vi "LEP_RV_PrepareLaunch.vi"(8 "error in (no error)":errorcluster, 10 "Enable debugging":bool, 11 "Commands":T1) -> (0 "error out":errorcluster, 2 "debug occurrence":refnum<k4>, 3 "output cluster":refnum<vi>)   [LabVIEW 2011]
doc: "Download and execute built VxWorks downloadable module and attach the LabVIEW Embedded debuger."
uses:
  LEP_RV_Commands.ctl
  <vilib>/Platform/EmbProject/utilities/Emb_Utility_AppAction.ctl
  LEP_RV_Config.ctl
panel:
  out "output cluster 2":T4 {"Config"."Constant Deallocation" items=["Out of Scope", "VI End", "Application End"]; "Config"."Constant Allocation" items=["First Use", "Containing Loop", "VI Initialization", "Application Initialization"]; "Config"."Target serial port" items=["0", "1", "2", "3"]; "Config"."Console output" items=["Processor status window", "Serial port"]; "Config"."Optimization" items=["Level 0 (-O0)", "Level 1 (-O1)", "Level 2 (-O2)", "Level 3 (-O3)"]; "Config"."Mode" items=["ARM-Mode", "Thumb-Mode"]; "Config"."Debug Options" items=["Use ULINK Debugger", "Use Simulator"]; "Config"."Debug Mode" items=["Instrumented (serial port)", "Instrumented (TCP/IP)", "Non-instrumented (JTAG/USB)"]}
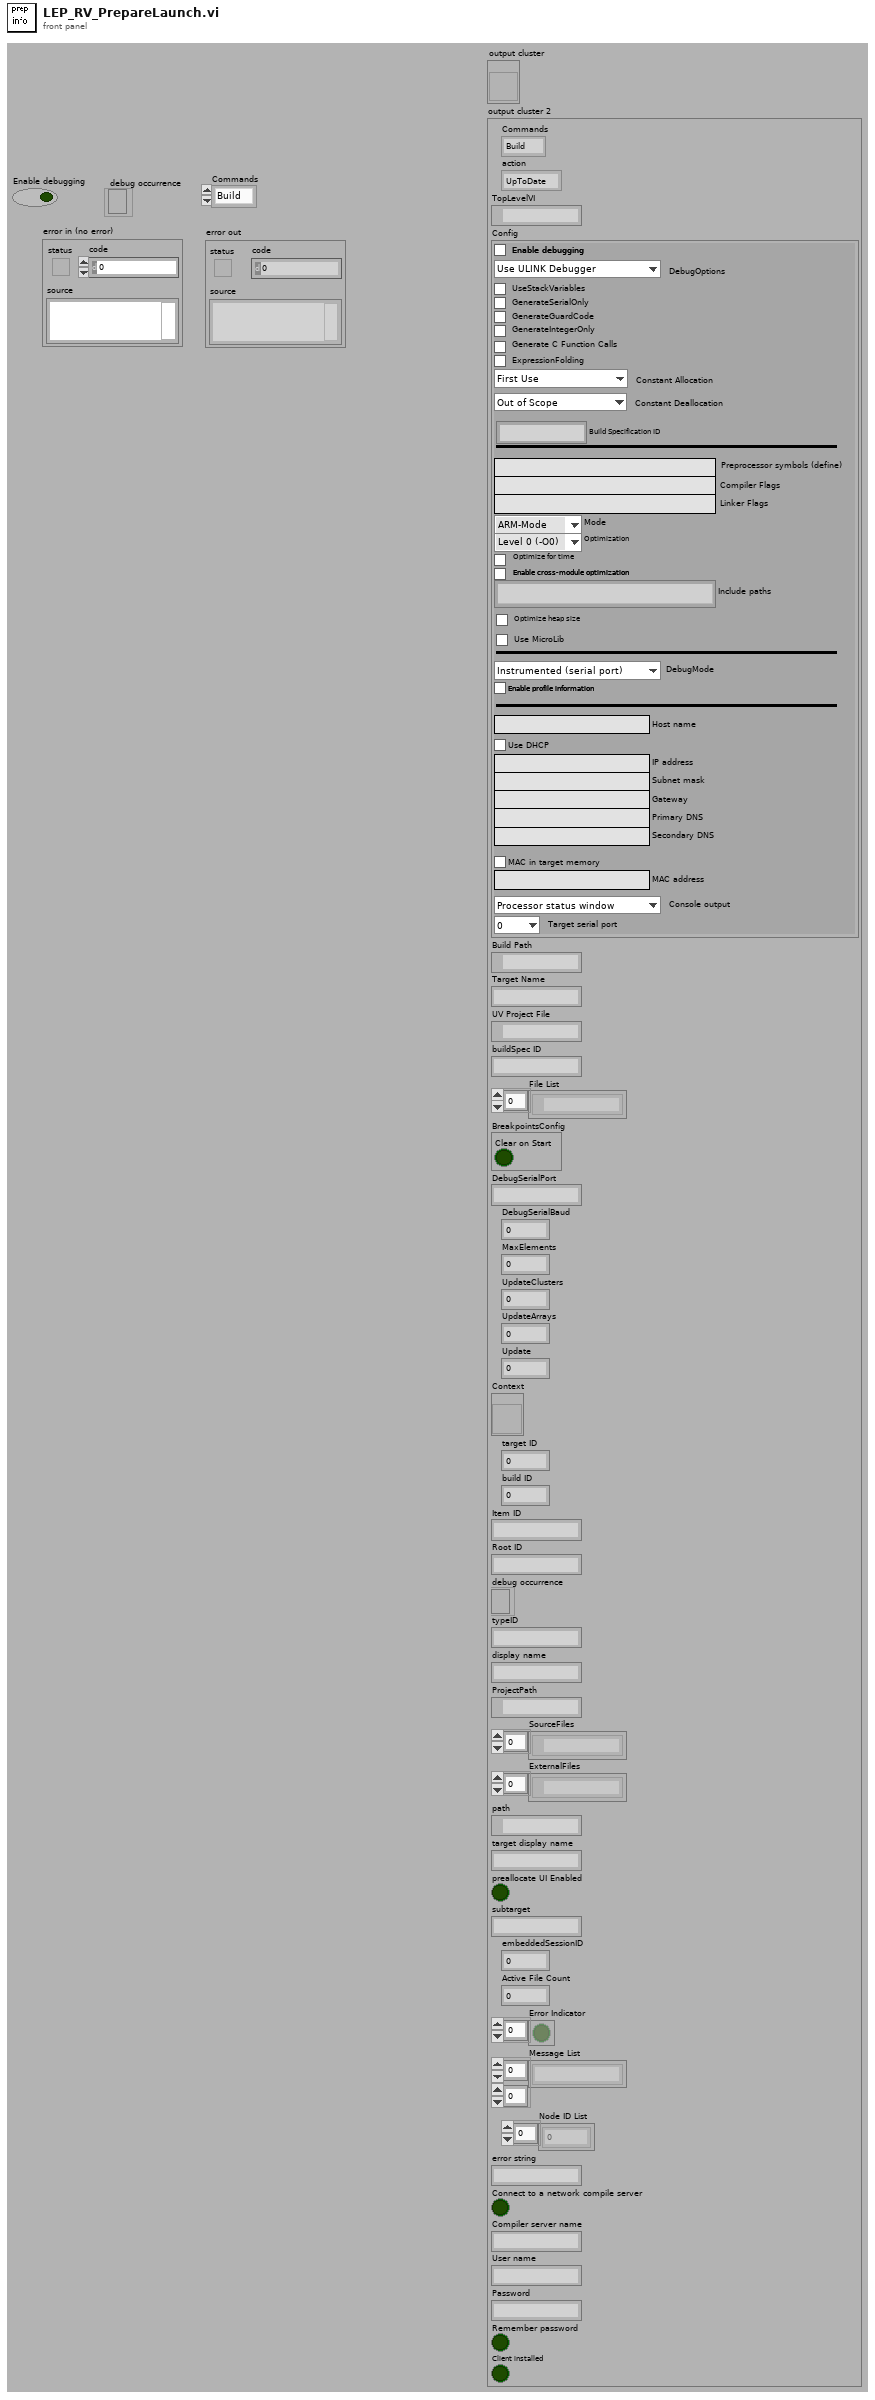
[diagram p1: front panel]
types:
  T1 = typedef "LEP_RV_Commands.ctl" = enum16{"Build", "Rebuild", "Run", "Debug", "Profile"}
  T2 = typedef "Emb_Utility_AppAction.ctl" = enum16{"UpToDate", "Build", "Cancel", "Error"}
  T3 = typedef "LEP_RV_Config.ctl" = cluster{"Enable debugging":bool, "Debug Options":u16, "Use stack variables":bool, "Generate serial only":bool, "Generate guard code":bool, "Generate Integer Only":bool, "Generate C Function Calls":bool, "ExpressionFolding":bool, "Constant Allocation":u16, "Constant Deallocation":u16, "Build Specification ID":string, "Preprocessor symbols (define)":string, "Compiler Flags":string, "Linker Flags":string, "Mode":u16, "Optimization":u16, "Optimize for time":bool, "Enable cross-module optimization":bool, "Include paths":path[], "Optimize heap size":bool, "Use MicroLib":bool, "Debug Mode":u16, "Enable profile information":bool, "Host name":string, "Use DHCP":bool, "IP address":string, "Subnet mask":string, "Gateway":string, "Primary DNS":string, "Secondary DNS":string, "MAC in target memory":bool, "MAC address":string, "Console output":u16, "Target serial port":u16}
  T4 = cluster{"Commands":T1, "action":T2, "TopLevelVI":path, "Config":T3, "Build Path":path, "Target Name":string, "UV Project File":path, "buildSpec ID":string, "File List":path[], "BreakpointsConfig":cluster{"Clear on Start":bool}, "DebugSerialPort":string, "DebugSerialBaud":u32, "MaxElements":u32, "UpdateClusters":u32, "UpdateArrays":u32, "Update":u32, "Context":refnum<vi>, "target ID":u32, "build ID":u32, "Item ID":string, "Root ID":string, "debug occurrence":refnum<k4>, "typeID":string, "display name":string, "ProjectPath":path, "SourceFiles":path[], "ExternalFiles":path[], "path":path, "target display name":string, "preallocate UI Enabled":bool, "subtarget":string, "embeddedSessionID":u32, "Active File Count":i32, "Error Indicator":bool[], "Message List":string[][], "Node ID List":i32[], "error string":string, "Connect to a network compile server":bool, "Compiler server name":string, "User name":string, "Password":string, "Remember password":bool, "Client installed":bool}
  T5 = enum16{"NoErr", "TopLevelVIErr", "EmptyTopLevelVIPath", "CGenErr", "CpySuppFilesErr", "ProjectInfoErr", "NoTopLevelVIErr", "CreateBuildFolderErr", "EmptyBuildFolderErr", "LoadConfigErr", "BildToolsErr", "CompileErr", "LinkError", "DebugInfoErr", "NotFoundErr", "AccessErr", "ExecErr", "UnknownErr"}
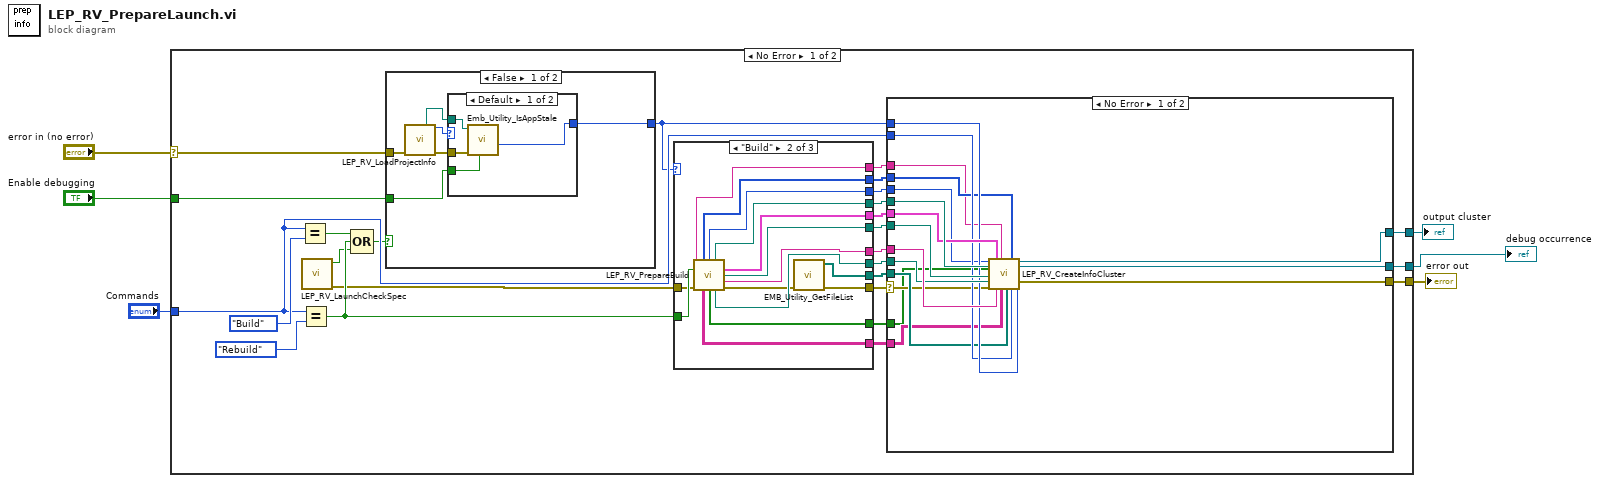
[diagram p0: block diagram]
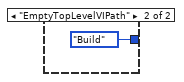
[diagram p2: hidden frame]
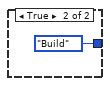
[diagram p3: hidden frame]
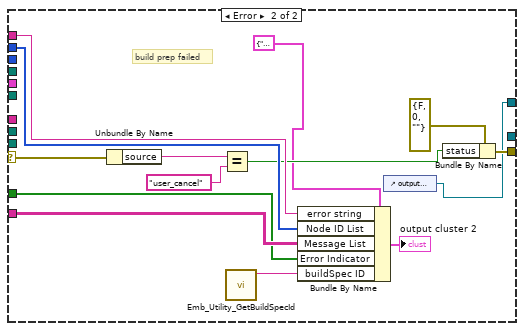
[diagram p4: hidden frame]
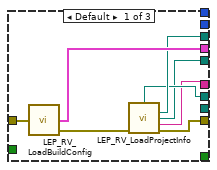
[diagram p5: hidden frame]
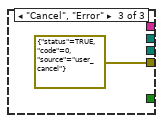
[diagram p6: hidden frame]
diagram:
  n1 = case shown="No Error" "error in (no error)" {
    selector: "error in (no error)" -> [w18 w100]
    tunnel: [w17 w100] -> w6
    tunnel: "Commands" -> [w30 _]
    tunnel: [w16 _] -> w3
    tunnel: "Enable debugging" -> [w15 _]
    tunnel: [w14 _] -> w1
    frame No Error {
      n2 = Equal?(x=w30, y=LEP_RV_Commands."Build") -> (x = y?=w27:bool)
      n3 = Equal?(x=w30, y=LEP_RV_Commands."Rebuild") -> (x = y?=w26:bool)
      n4 = call "LEP_RV_LaunchCheckSpec.vi"() -> ("error out"=w8:errorcluster, "OK"=w7:bool)  [unwired: 10 in]
      n5 = Compound Arithmetic op=OR(w27, w26, w7) -> (w28:bool)
      n6 = case shown="False" w28 {
        tunnel: w18 -> [w35 _]
        tunnel: [w34 Emb_Utility_AppAction."Build" ("action")] -> w25
        tunnel: w15 -> [w33 _]
        frame False {
          n7 = call "LEP_RV_LoadProjectInfo.vi"("error in (no error)"=w35) -> ("Executable File"=w38:path, "Status"=w36:T5, "error out"=w37:errorcluster)  [unwired: 1 in, 11 out]
          n8 = case shown="Default" w36 {
            tunnel: w37 -> [w42 _]
            tunnel: [w41 Emb_Utility_AppAction."Build" ("action")] -> w34
            tunnel: w38 -> [w40 _]
            tunnel: w33 -> [w39 _]
            frame Default {
              n9 = call <vilib>:"Emb_Utility_IsAppStale.vi"("debugging"=w39, "error in (no error)"=w42, "application path"=w40) -> ("action"=w41:T2)  [unwired: 3 in, 5 out]
            }
            frame "EmptyTopLevelVIPath" {
            }
          }
        }
        frame True {
        }
      }
      n10 = case shown="\"Build\"" w25 {
        tunnel: w26 -> [_ w98 _]
        tunnel: [w77 w90 errorcluster {"status"=TRUE, "code"=0, "source"="user_cancel"} ("error out")] -> w32
        tunnel: [w82 w97 _] -> w24
        tunnel: [w83 w96 _] -> w23
        tunnel: [w79 w95 _] -> w22
        tunnel: [w80 w94 _] -> w21
        tunnel: [w81 w93 _] -> w20
        tunnel: [_ w92 _] -> w19
        tunnel: [_ w89 _] -> w13
        tunnel: [_ w88 _] -> w10
        tunnel: [_ w87 _] -> w9
        tunnel: [_ w86 _] -> w11
        tunnel: [_ w85 _] -> w12
        tunnel: w8 -> [w76 w84 _]
        frame Default {
          n11 = call "LEP_RV_LoadBuildConfig.vi"("error in (no error)"=w76) -> ("Config"=w83:T3, "error out"=w78:errorcluster)  [unwired: 1 out]
          n12 = call "LEP_RV_LoadProjectInfo.vi"("error in (no error)"=w78) -> ("Project File"=w81:path, "TopLevelVIPath Out"=w82:path, "Build Path"=w79:path, "Target Name"=w80:string, "error out"=w77:errorcluster)  [unwired: 1 in, 9 out]
        }
        frame "Build" {
          n13 = call "LEP_RV_PrepareBuild.vi"("Rebuild"=w98, "error in (no error)"=w84) -> ("error string"=w85:string, "Node ID List"=w86:i32[], "Active File Count"=w89:i32, "TopLevelVI"=w97:path, "Config"=w96:T3, "Build Path"=w95:path, "Target Name"=w94:string, "Message List"=w87:string[][], "Error Indicator"=w88:bool[], "UV Project File"=w93:path, "error out"=w91:errorcluster)  [unwired: 2 in, 1 out]
          n14 = call <vilib>:"EMB_Utility_GetFileList.vi"("error in (no error)"=w91) -> ("error out"=w90:errorcluster, "File List"=w92:path[])  [unwired: 9 out]
        }
        frame "Cancel", "Error" {
        }
      }
      n15 = case shown="No Error" w32 {
        selector: w32 -> [w51 w70]
        tunnel: [w50 w65] -> w17
        tunnel: w30 -> [w55 _]
        tunnel: w25 -> [w56 _]
        tunnel: w24 -> [w61 _]
        tunnel: w23 -> [w60 _]
        tunnel: w22 -> [w59 _]
        tunnel: w21 -> [w58 _]
        tunnel: w20 -> [w57 _]
        tunnel: w19 -> [w54 _]
        tunnel: [w53 _] -> w16
        tunnel: [w52 w62] -> w14
        tunnel: w13 -> [w49 _]
        tunnel: w12 -> [w45 w73]
        tunnel: w11 -> [w48 w74]
        tunnel: w10 -> [w46 w72]
        tunnel: w9 -> [w47 w75]
        frame No Error {
          n16 = call "LEP_RV_CreateInfoCluster.vi"("Active File Count"=w49, "TopLevelVI"=w61, "Error Indicator"=w46, "Build Path"=w59, "UV Project File"=w57, "error IO"=w51, "Config"=w60, "Target Name"=w58, "error string"=w45, "Message List"=w47, "File List"=w54, "Node ID List"=w48, "Commands"=w55, "action"=w56) -> ("output cluster"=w52:refnum<vi>, "occurrence"=w53:refnum<k4>, "error out"=w50:errorcluster)  [unwired: 3 in]
        }
        frame Error {
          # "build prep failed"
          n17 = Unbundle By Name(w70) -> ("source"=w69:string)
          n18 = Equal?(x=w69, y="user_cancel") -> (x = y?=w66:bool)
          n19 = call <vilib>:"Emb_Utility_GetBuildSpecId.vi"() -> ("buildSpec ID"=w71:string)  [unwired: 1 in, 8 out]
          n20 = Bundle By Name(cluster=T4 {"Commands"=enum."Build", "action"=enum."UpToDate", "TopLevelVI"=path "", "Config"={"Enable debugging"=FALSE, "Debug Options"=0, "Use stack variables"=FALSE, "Generate serial only"=FALSE, "Generate guard code"=FALSE, "Generate Integer Only"=FALSE, "Generate C Function Calls"=FALSE, "ExpressionFolding"=FALSE, "Constant Allocation"=0, "Constant Deallocation"=0, "Build Specification ID"="", "Preprocessor symbols (define)"="", "Compiler Flags"="", "Linker Flags"="", "Mode"=0, "Optimization"=0, "Optimize for time"=FALSE, "Enable cross-module optimization"=FALSE, "Include paths"=[], "Optimize heap size"=FALSE, "Use MicroLib"=FALSE, "Debug Mode"=0, "Enable profile information"=FALSE, "Host name"="", "Use DHCP"=FALSE, "IP address"="", "Subnet mask"="", "Gateway"="", "Primary DNS"="", "Secondary DNS"="", "MAC in target memory"=FALSE, "MAC address"="", "Console output"=0, "Target serial port"=0}, "Build Path"=path "", "Target Name"="", "UV Project File"=path "", "buildSpec ID"="", "File List"=[], "BreakpointsConfig"={"Clear on Start"=FALSE}, "DebugSerialPort"="", "DebugSerialBaud"=0, "MaxElements"=0, "UpdateClusters"=0, "UpdateArrays"=0, "Update"=0, "Context"=refnum, "target ID"=0, "build ID"=0, "Item ID"="", "Root ID"="", "debug occurrence"=refnum, "typeID"="", "display name"="", "ProjectPath"=path "", "SourceFiles"=[], "ExternalFiles"=[], "path"=path "", "target display name"="", "preallocate UI Enabled"=FALSE, "subtarget"="", "embeddedSessionID"=0, "Active File Count"=0, "Error Indicator"=[], "Message List"=[], "Node ID List"=[], "error string"="", "Connect to a network compile server"=FALSE, "Compiler server name"="", "User name"="", "Password"="", "Remember password"=FALSE, "Client installed"=FALSE} ("output cluster"), "error string"=w73, "Node ID List"=w74, "Message List"=w75, "Error Indicator"=w72, "buildSpec ID"=w71) -> (→"output cluster 2":T4)
          n21 = control-ref of="output cluster 2"() -> (w62:refnum<vi>)
          n22 = Bundle By Name(cluster=errorcluster {"status"=FALSE, "code"=0, "source"=""} ("error out"), "status"=w66) -> (w65:errorcluster)
        }
      }
    }
    frame Error {
    }
  }
  "error out" <- w6
  "debug occurrence" <- w3
  "output cluster" <- w1
